vi "Controller Write PS Setpoints.vi"(0 "PS Setpoint Variables":refnum<k21>[](array[refnum]), 1 "PS Enable Variables":refnum<k21>[](array[refnum]), 2 "PS Setpoints":dbl[](array[numeric]), 3 "error in (no error)":errorcluster) -> (10 "error out":errorcluster)   [LabVIEW 2011, in "Controller VIs.lvlib"]
doc: "Writes PS Setpoints variables to the Actuation chassis."
uses:
  Controller VIs.lvlib
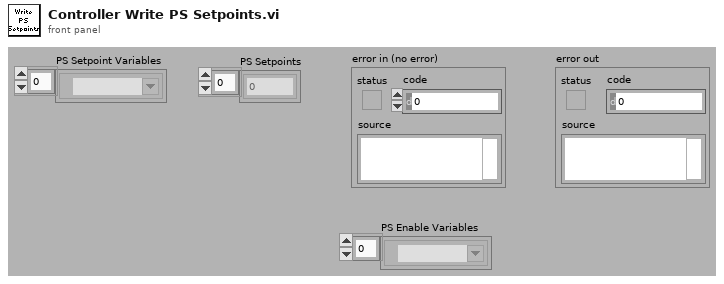
[diagram p1: front panel]
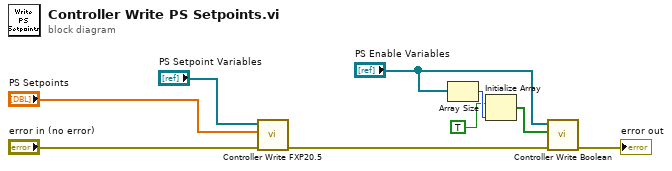
[diagram p0: block diagram]
diagram:
  n1 = call "Controller Write FXP20.5.vi"("Error In"="error in (no error)", "Values"="PS Setpoints", "Variables"="PS Setpoint Variables") -> ("Error Out"=w3:errorcluster)  [unwired: 8 in]
  n2 = Array Size(array="PS Enable Variables") -> (size(s)=w6:i32)
  n3 = Initialize Array(TRUE, w6) -> (w5:bool[])
  n4 = call "Controller Write Boolean.vi"("Error In"=w3, "Values"=w5, "Variables"="PS Enable Variables") -> ("Error Out"=→"error out":errorcluster)  [unwired: 8 in]
